vi "alinha_com_parede_odometria.vi"(5 "Line":i16(ring) items=["1", "2", "3", "4", "5", "6", "7", "8", "9", "10", "11", "12"], 8 "Text":string, 10 "NXT/EV3":T1) -> (0 "Numeric":dbl format="%#_13g", 2 "NXT/EV3 2":T1)   [LabVIEW 2016]
uses:
  <vilib>/NXT/Subs/LVHSConnector.ctl
  <vilib>/NXT/LegoClasses/BrickReference/BrickReference.lvclass
  <vilib>/NXT/Block Support/NXT_OutputPort.ctl
  <vilib>/NXT/Block Support/NXT_InputPort.ctl
  <vilib>/NXT/Dual Mode Library/Motors/ResetMotor.vi
  <vilib>/NXT/Dual Mode Library/Sensors/Touch_Pressed.vi
  <vilib>/NXT/NXTIO Xnodes/NXTIONodeSubVIs/NXTMoveMotors.vi
  <vilib>/NXT/Dual Mode Library/Motors/Rotation.vi
  <vilib>/NXT/Dual Mode Library/Display/drawText.vi
  <vilib>/NXT/Dual Mode Library/Display/drawNumber_float.vi
  <vilib>/NXT/NXTIO Xnodes/AddressXNode/NXTIOAddress.xnode
  <vilib>/NXT/NXTIO Xnodes/NXTIOXNode/NXTIO.xnode
panel:
  in  "KE 2":dbl=-0.0356
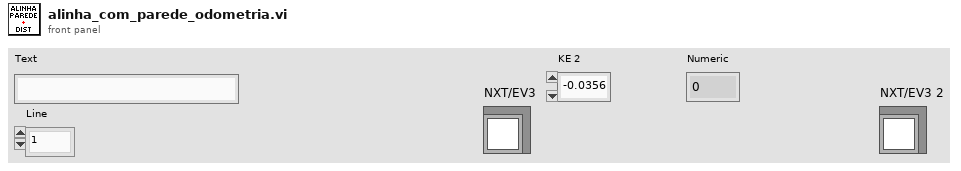
[diagram p1: front panel]
types:
  T1 = typedef "LVHSConnector.ctl" = refnum<class "BrickReference.lvclass">
  T2 = typedef "NXT_OutputPort.ctl" = u8
  T3 = typedef "NXT_InputPort.ctl" = u32
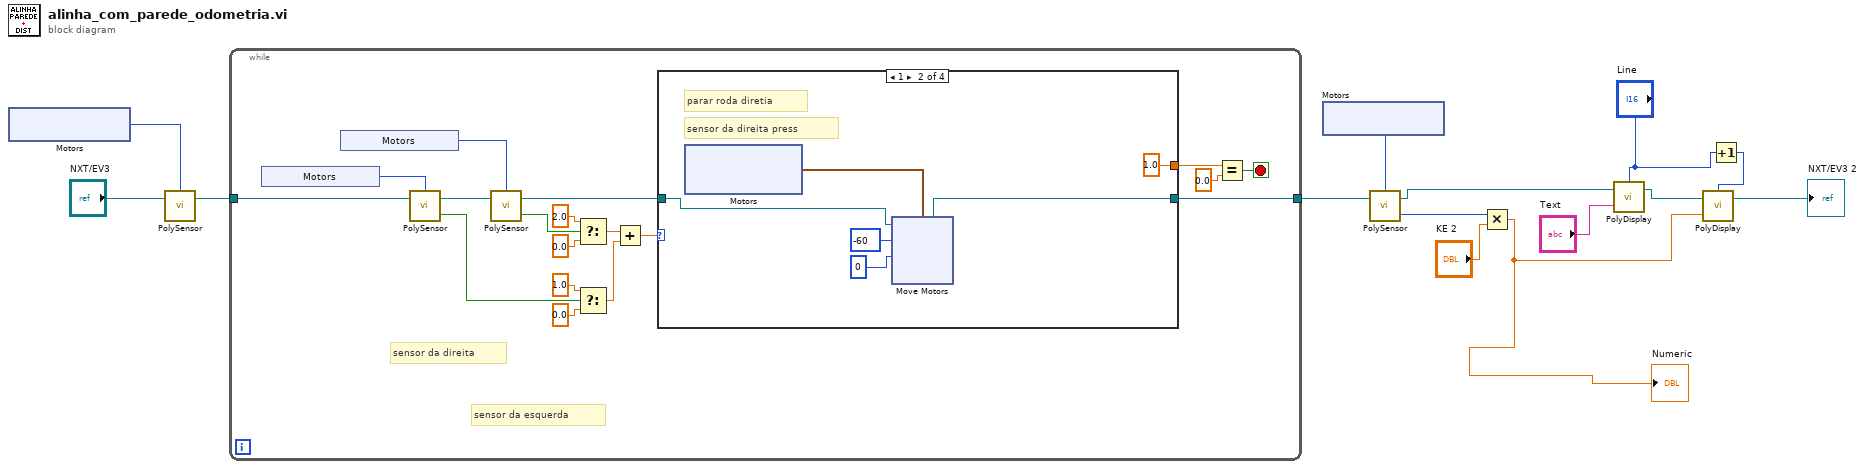
[diagram p0: block diagram]
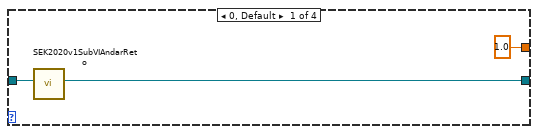
[diagram p2: hidden frame]
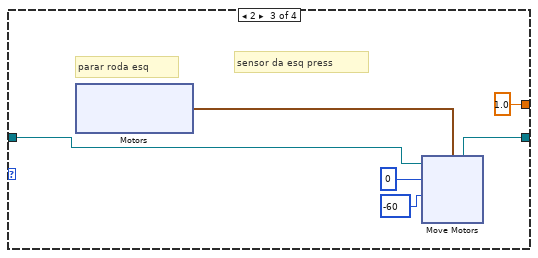
[diagram p3: hidden frame]
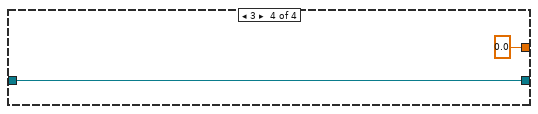
[diagram p4: hidden frame]
diagram:
  n1 = xnode "Motors"() -> ("Motor"=w14:T2)
  n2 = call-poly <vilib>:"PolySensor.vi"("NXT/EV3"="NXT/EV3", "Port (All Ports)"=w14) -> ("NXT/EV3"=w10:T1)  [unwired: 2 out]
  n3 = while {
    tunnel: w10 -> [w15]
    tunnel: [w25] -> w12
    stop <- w22 stop-if-true
    # "sensor da esquerda"
    # "sensor da direita"
    n4 = xnode "Motors"() -> ("Sensor"=w21:T3)
    n5 = xnode "Motors"() -> ("Sensor"=w20:T3)
    n6 = call-poly <vilib>:"PolySensor.vi"("NXT/EV3"=w15, "Port (Port 1)"=w21) -> ("Yes / No"=w31:bool, "NXT/EV3"=w32:T1)  [unwired: 1 in]
    n7 = call-poly <vilib>:"PolySensor.vi"("NXT/EV3"=w32, "Port (Port 1)"=w20) -> ("Yes / No"=w26:bool, "NXT/EV3"=w16:T1)  [unwired: 1 in]
    n8 = Select(t=2.0, s=w26, f=0.0 ("t")) -> (s? t:f=w19:dbl)
    n9 = Select(t=1.0, s=w31, f=0.0 ("t")) -> (s? t:f=w18:dbl)
    n10 = Add(x=w19, y=w18) -> (x+y=w17:dbl)
    n11 = case shown="1" w17 {
      tunnel: w16 -> [w36 w40 w55 w69]
      tunnel: [w37 w39 w54 w69] -> w25
      tunnel: [1.0 ("t") 1.0 ("t") 1.0 ("t") 0.0 ("t")] -> w24
      frame 0, Default {
        n12 = call "SEK2020v1SubVIAndarReto.vi"("NXT/EV3"=w36) -> ("NXT/EV3 2"=w37:T1)  [unwired: 9 in]
      }
      frame 1 {
        # "parar roda diretia"
        # "sensor da direita press"
        n13 = xnode "Motors"() -> ("Motor"=w41:cluster{"Port":T2, "Port":T2})
        n14 = xnode "Move Motors"("Power/Speed 2"=i8 0, "Power/Speed 1"=i8 -60, "Motors"=w41, "NXT/EV3"=w40) -> ("NXT/EV3"=w39:T1)
      }
      frame 2 {
        # "parar roda esq"
        # "sensor da esq press"
        n15 = xnode "Motors"() -> ("Motor"=w58:cluster{"Port":T2, "Port":T2})
        n16 = xnode "Move Motors"("Power/Speed 2"=i8 -60 ("Power/Speed 1"), "Power/Speed 1"=i8 0 ("Power/Speed 2"), "Motors"=w58, "NXT/EV3"=w55) -> ("NXT/EV3"=w54:T1)
      }
      frame 3 {
      }
    }
    n17 = Equal?(x=w24, y=0.0 ("t")) -> (x = y?=w22:bool)
  }
  n18 = xnode "Motors"() -> ("Motor"=w13:T2)
  n19 = call-poly <vilib>:"PolySensor.vi"("NXT/EV3"=w12, "Port (Port A)"=w13) -> ("Angle of Rotation"=w7:i32, "NXT/EV3"=w6:T1)  [unwired: 1 out]
  n20 = Multiply(x=w7, y="KE 2") -> (x*y=w1:dbl)
  "Numeric" <- w1
  n21 = call-poly <vilib>:"PolyDisplay.vi"("Text"="Text", "NXT/EV3"=w6, "Line"="Line") -> ("NXT/EV3"=w5:T1)  [unwired: 1 in]
  n22 = Increment(x="Line") -> (x+1=w2:i16)
  n23 = call-poly <vilib>:"PolyDisplay.vi"("number"=w1, "NXT/EV3"=w5, "Line"=w2) -> ("NXT/EV3"=→"NXT/EV3 2":T1)  [unwired: 1 in]
